vi "Read Glyphs from  File.vi"(6 "File Name":string="Glyphs.bin", 7 "Path":T1=enum."Glyphs", 8 "error in (no error)":errorcluster) -> (0 "error out":errorcluster, 3 "Graphics":T2[](array[typedef]))   [LabVIEW 2020]
uses:
  vi.lib/LabVIEW Icon API/lv_icon/lv_icon.lvlib
  Controls/Path&Icon.ctl
  vi.lib/LabVIEW Icon API/lv_icon/Controls/Pathes.ctl
panel:
  in  "?":T2[](array[typedef])
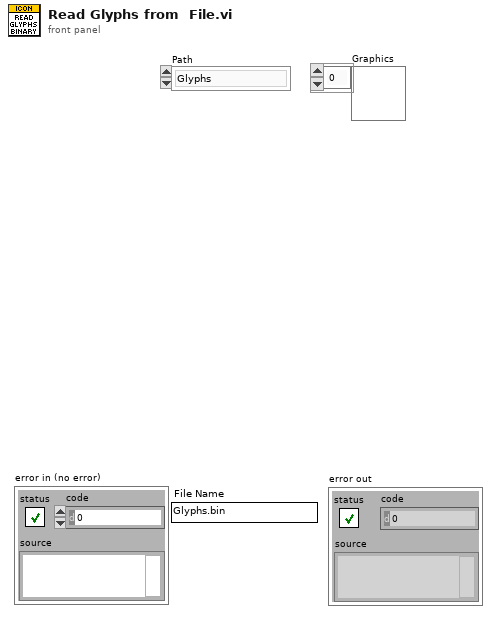
[diagram p1: front panel]
types:
  T1 = typedef "Pathes.ctl" = enum16{"Root Path", "Icon Templates", "Icon Templates VI", "Icon Templates Lib", "Glyphs"}
  T2 = typedef "Path&Icon.ctl" = cluster{"Rectangle":cluster{"left":i16, "top":i16, "right":i16, "bottom":i16}, "Path":path, "Image":picture, "Filter":string, "FileName":string}
  T3 = enum16{"open", "replace", "create", "open or create", "replace or create", "replace or create with confirmation"}
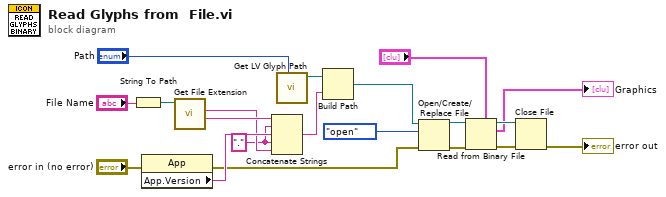
[diagram p0: block diagram]
diagram:
  w1 = "." ("string")
  n1 = String To Path(string="File Name") -> (path=w4:path)
  n2 = property class="App"(error in="error in (no error)") -> (error out=w8:errorcluster, "App.Version"=w10:string)  [unwired: 1 in, 1 out]
  n3 = call <vilib>:"Get File Extension.vi"("file"=w4) -> ("filename without extension"=w3:string, "lowercase file extension"=w2:string)  [unwired: 1 in, 8 out]
  n4 = Concatenate Strings(w3, w1, w10, w1, w2) -> (w7:string)
  n5 = call "Get LV Glyph Path.vi"("Path"="Path") -> ("Requested Path"=w19:path)  [unwired: 2 in, 8 out]
  n6 = Build Path(base path=w19, name or relative path=w7) -> (appended path=w18:path)
  n7 = Open/Create/Replace File(file path (use dialog)=w18, error in=w8, operation (0:open)=T3."open") -> (refnum out=w16:refnum<file>, error out=w17:errorcluster)  [unwired: 1 in, 3 out]
  n8 = Read from Binary File(5:"?", 8:w17, 11:w16) -> (0:w15:errorcluster, 2:→"Graphics":T2[], 3:w14:refnum<file>)  [unwired: 4 out]
  n9 = Close File(refnum=w14, error in=w15) -> (error out=→"error out":errorcluster)  [unwired: 1 out]
